vi "Actor Core.vi"(8 "error in":errorcluster, 11 "Chart Actor in":refnum<class "Chart Actor.lvclass">) -> (0 "error out":errorcluster, 3 "Actor out":refnum<class "Actor.lvclass">)   [LabVIEW 2021, in "Chart Actor.lvlib" / "Chart Actor.lvclass"]
doc: "(<B>Filename</B>: Actor Framework.lvlib:Actor.lvclass:Actor Core.vi)\n\nReceives messages to the actor, reacts to them, and initiates any error handling that may shut the actor down.\n\nDescendant classes may override this VI to append parallel tasks for the actor to complete while it handles messages. Overrides use the Call Parent Class Method node."
uses:
  Chart Actor.lvclass
  <vilib>/ActorFramework/Actor/Actor.lvclass
  Chart Actor.lvclass/Chart Actor.ctl
panel:
  out "element":dbl
  out "Waveform Chart":waveform(dbl)(graph)
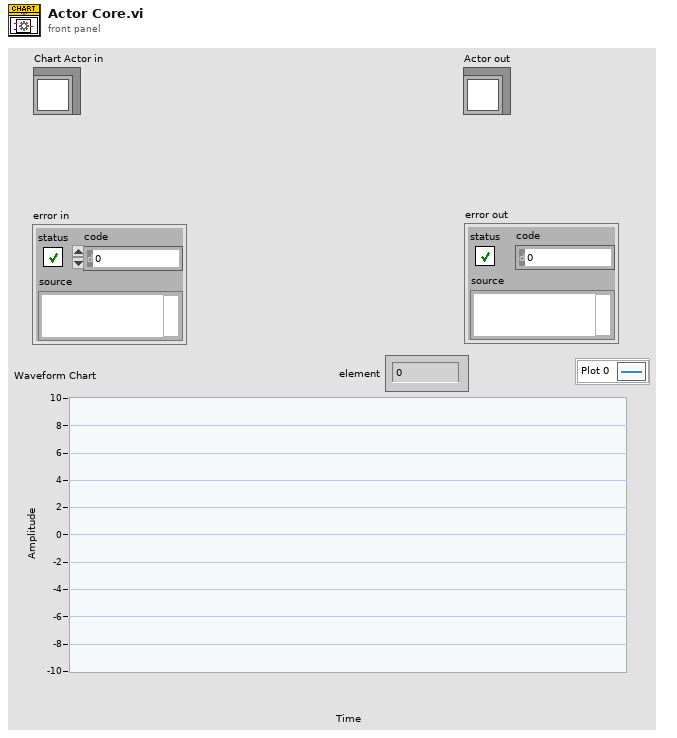
[diagram p1: front panel]
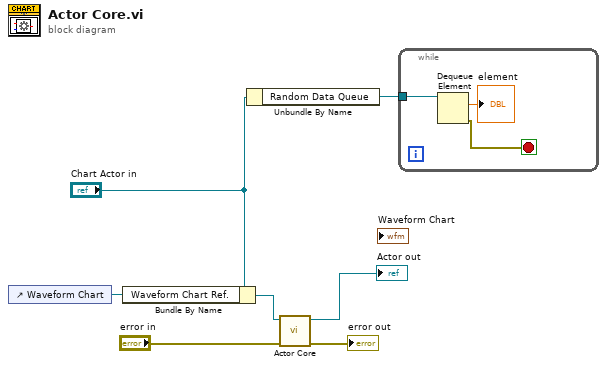
[diagram p0: block diagram]
diagram:
  n1 = control-ref of="Waveform Chart"() -> (w4:refnum<vi>)
  n2 = Bundle By Name(cluster="Chart Actor in", "Waveform Chart Ref."=w4) -> (w3:refnum<class "Chart Actor.lvclass">)
  n3 = Unbundle By Name("Chart Actor in") -> ("Random Data Queue"=w1:refnum<queue>)
  n4 = call-parent "Actor Core.vi"("error in"="error in", "Actor in"=w3) -> ("error out"=→"error out":errorcluster, "Actor out"=→"Actor out":refnum<class "Actor.lvclass">)  [unwired: 8 in]
  n5 = while {
    tunnel: w1 -> [w10]
    stop <- w9 stop-if-true
    n6 = Dequeue Element(queue=w10) -> (element=→"element":dbl, error out=w9:errorcluster)  [unwired: 2 in, 2 out]
  }
